vi "check syntax_core.vi"(8 "error in (no error)":errorcluster caption="에러 입력(에러 없음)", 11 "Script Line_i2c sr 입력":refnum<class "Script Line_i2c sr.lvclass">) -> (0 "error out":errorcluster caption="에러 출력", 3 "Script Line_i2c sr 출력":refnum<class "Script Line_i2c sr.lvclass">)   [LabVIEW 2020, in "Script Line_i2c sr.lvclass"]
uses:
  Script Line_i2c sr.lvclass
  Script Line/Script Line.lvclass/Script Line.ctl
  Script Line_i2c/Script Line_i2c.lvclass/Script Line_i2c.ctl
  Script Line_i2c/Accessors/Write slv.vi
  Script Line_i2c/Accessors/Write reg.vi
  Script Line_i2c/Accessors/Write reg addr byte.vi
  Script Line_i2c/Accessors/Write size.vi
  Script Line/Accessors/Read parameter.vi
  Script Line/Accessors/Read parameter string index.vi
  Script Line/Script Line.lvclass
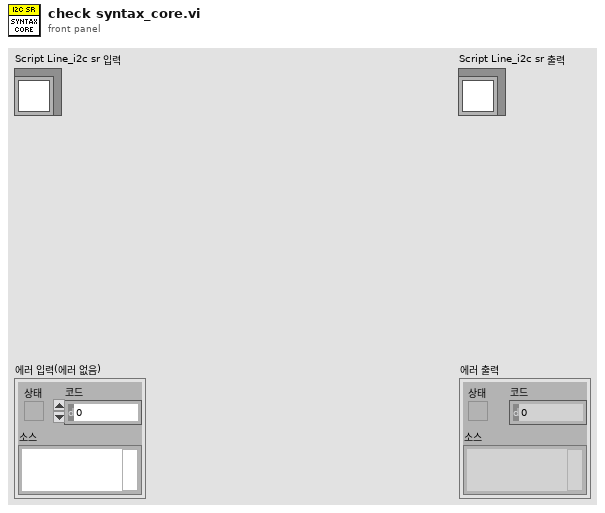
[diagram p1: front panel]
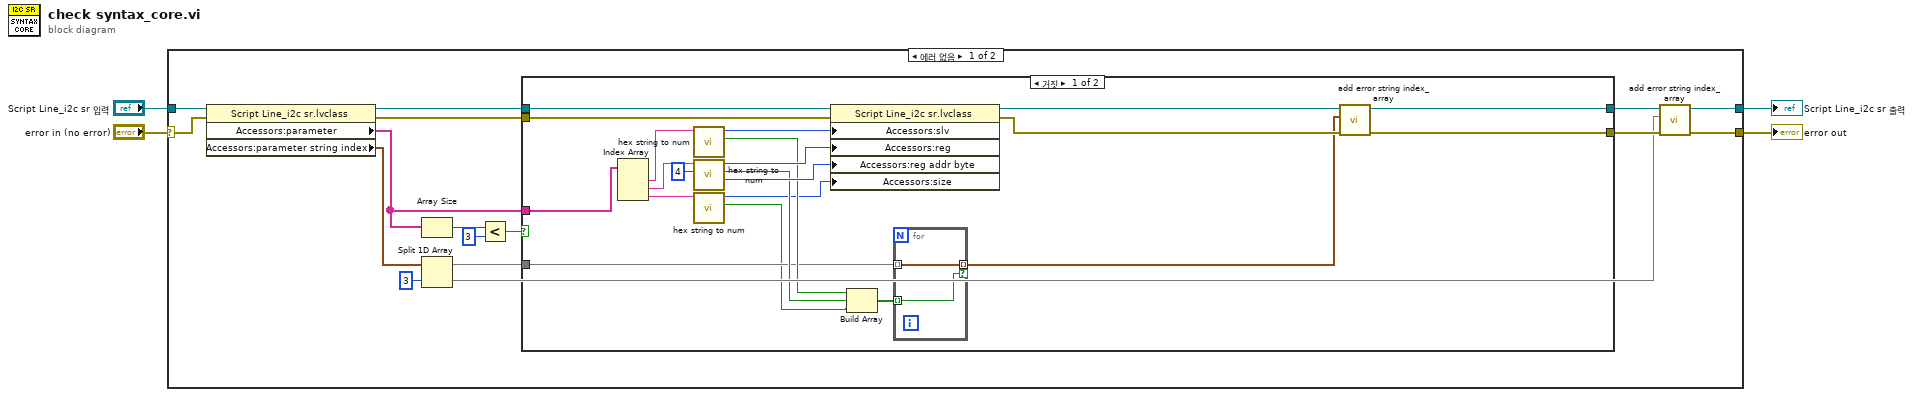
[diagram p0: block diagram]
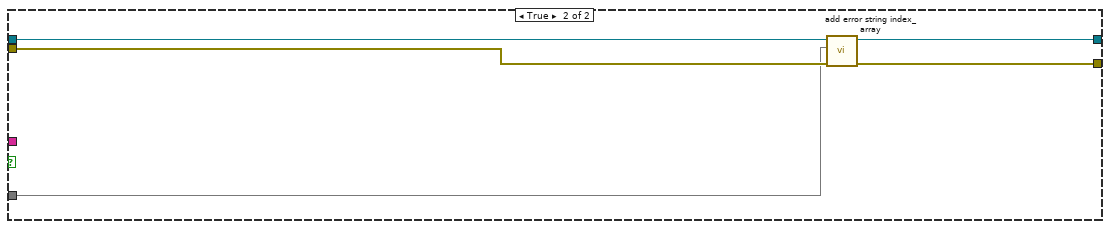
[diagram p2: hidden frame]
diagram:
  n1 = case shown="에러 없음" "error in (no error)" {
    selector: "error in (no error)" -> [w19 w50]
    tunnel: [w8 w50] -> w2
    tunnel: [w6 w49] -> w3
    tunnel: "Script Line_i2c sr 입력" -> [w20 w49]
    frame No Error {
      n2 = property class="Script Line_i2c sr.lvclass"(reference=w20, error in=w19) -> (reference out=w14:refnum<class "Script Line_i2c sr.lvclass">, error out=w13:errorcluster, "Accessors:parameter"=w15:string[], "Accessors:parameter string index"=w11:cluster{"start":u32, "end":u32}[])
      n3 = Array Size(array=w15) -> (size(s)=w18:i32)
      n4 = Split 1D Array(array=w11, index=3 ("인덱스")) -> (first subarray=w10:cluster{"start":u32, "end":u32}[], second subarray=w5:cluster{"start":u32, "end":u32}[])
      n5 = Less?(x=w18, y=3) -> (x < y?=w16:bool)
      n6 = case shown="거짓" w16 {
        tunnel: w15 -> [w21 _]
        tunnel: w10 -> [w23 w44]
        tunnel: w14 -> [w40 w46]
        tunnel: w13 -> [w41 w48]
        tunnel: [w24 w47] -> w12
        tunnel: [w25 w45] -> w7
        frame False {
          n7 = Index Array(array=w21) -> (element #1=w32:string, element #2=w33:string, element #3=w34:string)  [unwired: 3 in]
          n8 = call "hex string to num.vi"("string"=w32) -> ("error"=w30:bool, "num"=w35:u32)  [unwired: 7 in, 2 out]
          n9 = call "hex string to num.vi"("max byte (1)"=u8 4, "string"=w33) -> ("byte"=w38:u8, "error"=w29:bool, "num"=w39:u32)  [unwired: 6 in, 1 out]
          n10 = call "hex string to num.vi"("string"=w34) -> ("error"=w22:bool, "num"=w27:u32)  [unwired: 7 in, 2 out]
          n11 = property class="Script Line_i2c sr.lvclass"(reference=w40, error in=w41, "Accessors:slv"=w35, "Accessors:reg"=w39, "Accessors:reg addr byte"=w38, "Accessors:size"=w27) -> (reference out=w37:refnum<class "Script Line_i2c sr.lvclass">, error out=w36:errorcluster)
          n12 = Build Array(w30, w29, w22) -> (w28:bool[])
          n13 = for {
            tunnel: w23 -> [w43] mode=indexing
            tunnel: [w43] -> w26 mode=indexing if=w42
            tunnel: w28 -> [w42] mode=indexing
          }
          n14 = call "add error string index_array.vi"("error in (no error)"=w36, "index_array"=w26, "Script Line 입력"=w37) -> ("error out"=w24:errorcluster, "Script Line 출력"=w25:refnum<class "Script Line_i2c sr.lvclass">)  [unwired: 7 in]
        }
        frame True {
          n15 = call "add error string index_array.vi"("error in (no error)"=w48, "index_array"=w44, "Script Line 입력"=w46) -> ("error out"=w47:errorcluster, "Script Line 출력"=w45:refnum<class "Script Line_i2c sr.lvclass">)  [unwired: 7 in]
        }
      }
      n16 = call "add error string index_array.vi"("error in (no error)"=w12, "index_array"=w5, "Script Line 입력"=w7) -> ("error out"=w8:errorcluster, "Script Line 출력"=w6:refnum<class "Script Line_i2c sr.lvclass">)  [unwired: 7 in]
    }
    frame Error {
    }
  }
  "error out" <- w2
  "Script Line_i2c sr 출력" <- w3
